vi "play-analyze-z-axis-agilent.vi"() -> ()   [LabVIEW 2015]
uses:
  <vilib>/userdefined/High Color/nirio_resource_hc.ctl
  <vilib>/FPGAPlugInAG/cRIO-9082/niLvFpga_Open_cRIO-9082.vi
  <vilib>/rvi/interface/common/dynamic/niFpgaDynamicAddResources.vi
  <vilib>/FPGAPlugInAG/Dynamic/niLvFpga_Reset_Dynamic.vi
  <vilib>/rvi/interface/common/niFpgaWaitOnOcc.vi
  <vilib>/Utility/error.llb/Error Cluster From Error Code.vi
  <vilib>/rvi/errors/niLvFpgaAdjustHostInterfaceError.vi
  <vilib>/FPGAPlugInAG/Dynamic/niLvFpga_Run_Dynamic.vi
  <vilib>/Utility/file.llb/Write Delimited Spreadsheet (DBL).vi
  <vilib>/FPGAPlugInAG/Dynamic/niLvFpga_Close_Dynamic.vi
  <vilib>/rvi/interface/nirviOpenFPGA/nirviOpenFPGA.xnode
  FPGA Bitfiles/afmimagingcontro_FPGATargetSPARTA_analyze-z-axis-a_s0ep9mccPBQ.lvbitx
  <vilib>/rvi/interface/nirviMethod/nirviMethod.xnode
  <vilib>/rvi/interface/nirviReadWriteControl/nirviReadWriteControl.xnode
  <vilib>/rvi/interface/nirviCloseFPGA/nirviCloseFPGA.xnode
  <vilib>/rvi/errors/niLvFpgaMergeErrorWithErrorCode.vi
  <vilib>/FPGAPlugInAG/Dynamic/niLvFpga_ReadFifo_Dynamic.vi
  <vilib>/rvi/interface/Simulation/niFpgaSimulationCallBeginRW.vi
  <vilib>/FPGAPlugInAG/Dynamic/niLvFpga_ConfigureFifo_Dynamic.vi
  NiFpgaLv.dll
panel:
  in  "nsamps":i32
  out "Waveform Graph":dbl[](graph)
  in  "outputData BOTH":path=path "C:/Users/arnold/Documents/labview/afm_imaging/data/analyze-z-axis-PIon.csv"
  out "y iter":i32
  out "size(s)":i32
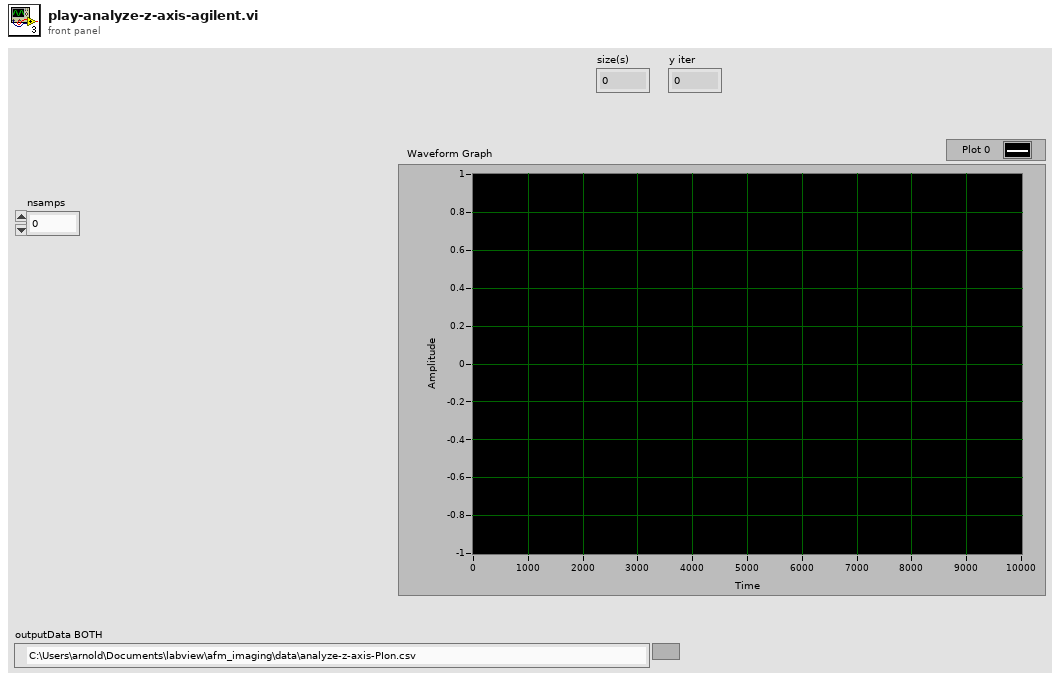
[diagram p1: front panel]
types:
  T1 = typedef "nirio_resource_hc.ctl" = tag
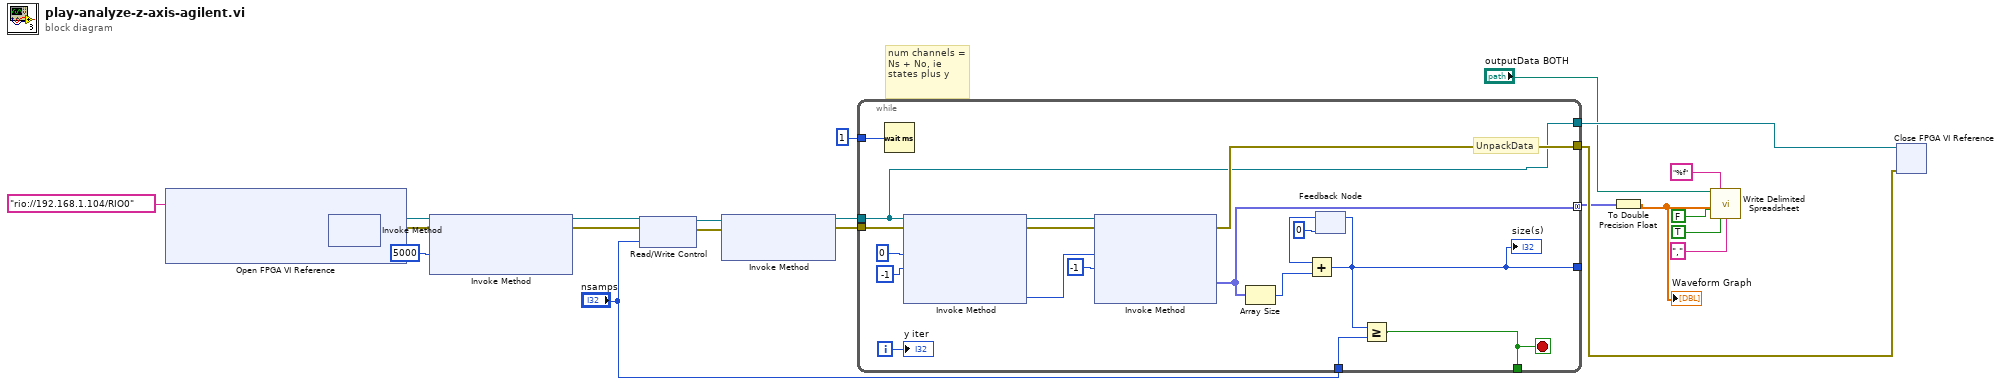
[diagram p0: block diagram]
diagram:
  # "num channels = Ns + No, ie states plus y"
  n1 = xnode "Open FPGA VI Reference"("resource name"=T1 "rio://192.168.1.104/RIO0") -> ("FPGA VI Reference Out"=w20:refnum<k20>, "error out"=w19:errorcluster)  [unwired: 1 in]
  n2 = xnode "Invoke Method"("FPGA VI Reference In"=w20, "error in"=w19) -> ("FPGA VI Reference Out"=w16:refnum<k20>, "error out"=w15:errorcluster)
  n3 = xnode "Invoke Method"("FPGA VI Reference In"=w16, "error in"=w15, "Requested Depth"=5000) -> ("FPGA VI Reference Out"=w14:refnum<k20>, "error out"=w13:errorcluster)  [unwired: 1 out]
  n4 = xnode "Read/Write Control"("FPGA VI Reference In"=w14, "error in"=w13, "nsamps"="nsamps") -> ("FPGA VI Reference Out"=w11:refnum<k20>, "error out"=w12:errorcluster)
  n5 = xnode "Invoke Method"("FPGA VI Reference In"=w11, "error in"=w12) -> ("FPGA VI Reference Out"=w10:refnum<k20>, "error out"=w17:errorcluster)  [unwired: 1 in]
  n6 = while {
    tunnel: 1 -> [w41]
    tunnel: w10 -> [w25]
    tunnel: w17 -> [w28]
    tunnel: [w34] -> w8
    tunnel: [w25] -> w22
    tunnel: [w31] -> w2 mode=concatenating
    tunnel: [w26] -> _
    tunnel: "nsamps" -> [w27]
    tunnel: [w24] -> _
    i -> [w33]
    stop <- w24 stop-if-true
    # "UnpackData"
    n7 = Wait (ms)(milliseconds to wait=w41) -> ()  [unwired: 1 out]
    n8 = xnode "Invoke Method"("FPGA VI Reference In"=w25, "error in"=w28, "Number of Elements"=0 ("Timeout (ms)"), "Timeout (ms)"=-1) -> ("FPGA VI Reference Out"=w37:refnum<k20>, "error out"=w38:errorcluster, "Elements Remaining"=w32:u32)  [unwired: 1 out]
    n9 = xnode "Invoke Method"("FPGA VI Reference In"=w37, "error in"=w38, "Number of Elements"=w32, "Timeout (ms)"=-1) -> ("error out"=w34:errorcluster, "Data"=w31:fxp<+/-,16,5>[])  [unwired: 2 out]
    n10 = Array Size(array=w31) -> (size(s)=w30:i32)
    n11 = feedback #1(0) -> (w29:i32)
    n12 = Add(x=w29, y=w30) -> (x+y=w26:i32)
    "size(s)" <- w26
    n13 = feedback-in #1(w26) -> ()
    n14 = Greater Or Equal?(x=w26, y=w27) -> (x >= y?=w24:bool)
    "y iter" <- w33
  }
  n15 = To Double Precision Float(number=w2) -> (double precision float=w3:dbl[])
  "Waveform Graph" <- w3
  n16 = call-poly <vilib>:"Write Delimited Spreadsheet.vi"("file path (dialog if empty)"="outputData BOTH", "format (%.3f)"="%f", "1D data"=w3, "append to file? (F)"=FALSE, "transpose? (F)"=TRUE, "delimiter (\\t)"=",") -> ()  [unwired: 8 in, 2 out]
  n17 = xnode "Close FPGA VI Reference"("FPGA VI Reference In"=w22, "error in"=w8) -> ()  [unwired: 1 out]
